vi "labview-quick-visualization.vi"   [LabVIEW 2020]
doc: "This example connects to nominal and ingests a single sample data point under a specified dataset. This should be used as a starting point for rapid data upload tasks.\n\nRequires:\nDataset RID\nAPI token\nSee client prerequisites for instructions on getting these values"
uses:
  Nominal Client/Nominal Client.lvclass/Nominal Client.ctl
  User/User.lvclass
  Nominal Client/Nominal Client.lvclass
  nominal types/workspace/workspace.lvclass
  submodules/reqwest-labview/lv-src/reqwest/reqwest.lvclass
  <vilib>/JDP Science/JSONtext/LVClass Serializer/JSONtext LVClass Serializer.lvclass
  nominal types/properties/properties.lvclass
  1ad2d2bf-605a-4f93-993e-8646e54caeef.vi
  255159e9-1e8d-4e07-9c25-a8834b7b3251.vi
  f949a3b6-5835-49af-8d06-1efcbc58f81d.vi
types:
  T1 = cluster{"Channel":string, "Points":cluster{"UNIX Timestamp":cluster{"Seconds":i32, "Nanoseconds":i32}, "Value":dbl}[]}[]
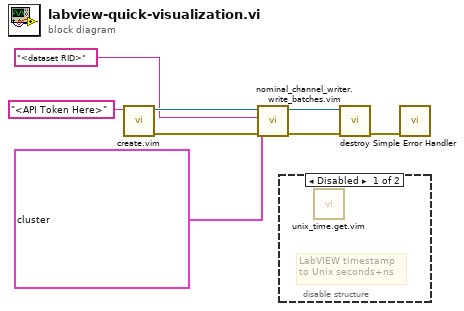
[diagram p0: block diagram]
diagram:
  n1 = call "create.vim"("API Token (string or path)"="<API Token Here>") -> ("error out"=w7:errorcluster, "Nominal Client"=w6:refnum<class "Nominal Client.lvclass">)  [unwired: 8 in, 1 out]
  n2 = call "nominal_channel_writer.write_batches.vim"("error in"=w7, "batches"=T1 [{"Channel"="voltage", "Points"=[{"UNIX Timestamp"={"Seconds"=1791319025, "Nanoseconds"=44529438}, "Value"=12.1}]}], "Data Source RID"="<dataset RID>" ("Dataset RID"), "Nominal Client in"=w6) -> ("error out"=w4:errorcluster, "Nominal Client out"=w5:refnum<class "Nominal Client.lvclass">)  [unwired: 5 in, 1 out]
  n3 = disable-structure shown="Disabled" {
    frame Disabled {
      # "LabVIEW timestamp\nto Unix seconds+ns"
      n4 = call "unix_time.get.vim"() -> ()  [unwired: 11 in, 1 out]
    }
    frame Enabled {
    }
  }
  n5 = call "destroy.vi"("error in"=w4, "Nominal Client"=w5) -> ("error out"=w1:errorcluster)  [unwired: 9 in]
  n6 = call <vilib>:"Simple Error Handler.vi"("error in (no error)"=w1) -> ()  [unwired: 4 in, 5 out]
